vi "Measurement Done.vi"(6 "Array of Hardware":refnum<class "Hardware.lvclass">[](array[class]), 8 "error in (no error)":errorcluster, 9 "Measurement Name":string, 10 "GUID":string, 11 "Controller in":refnum<class "Controller.lvclass">) -> (0 "error out":errorcluster, 3 "Controller out":refnum<class "Controller.lvclass">)   [LabVIEW 2026, in "Controller Actor.lvlib" / "Controller.lvclass"]
uses:
  Controller.lvclass
  Hardware/Hardware.lvclass
  Hardware/Hardware.lvclass/Hardware.ctl
  <vilib>/Utility/LVClass/Get LV Class Path.vi
  <userlib>/_OpenG.lib/file/file.llb/Strip Path Extension__ogtk.vi
  <userlib>/_OpenG.lib/file/file.llb/Strip Path Extension - String__ogtk.vi
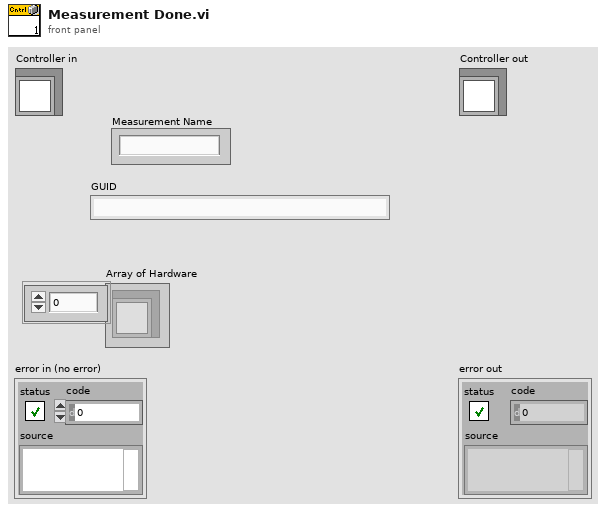
[diagram p1: front panel]
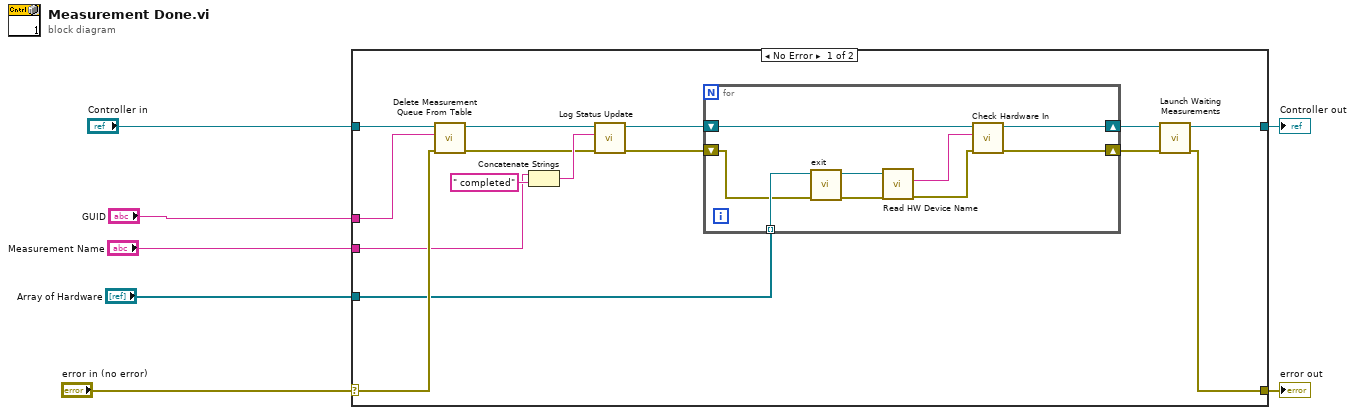
[diagram p0: block diagram]
diagram:
  n1 = case shown="No Error" "error in (no error)" {
    selector: "error in (no error)" -> [w12 w33]
    tunnel: [w11 w33] -> w6
    tunnel: [w21 w32] -> w4
    tunnel: "Controller in" -> [w15 w32]
    tunnel: "GUID" -> [w16 _]
    tunnel: "Measurement Name" -> [w10 _]
    tunnel: "Array of Hardware" -> [w9 _]
    frame No Error {
      n2 = call "Delete Measurement Queue From Table.vi"("error in (no error)"=w12, "Unique Identifier"=w16, "Controller in"=w15) -> ("error out"=w8:errorcluster, "Controller out"=w18:refnum<class "Controller.lvclass">)  [unwired: 7 in]
      n3 = Concatenate Strings(w10, " completed" ("string")) -> (w19:string)
      n4 = call-dynamic "Log Status Update.vi"("error in (no error)"=w8, "String"=w19, "Controller in"=w18) -> ("error out"=w14:errorcluster, "Controller out"=w17:refnum<class "Controller.lvclass">)  [unwired: 7 in]
      n5 = for {
        shift-right: [w30] -> w22
        shift-left: w17 -> [w31]
        shift-right: [w29] -> w13
        shift-left: w14 -> [w24]
        tunnel: w9 -> [w27] mode=indexing
        n6 = call "exit.vi"("error in (no error)"=w24, "Hardware in"=w27) -> ("error out"=w25:errorcluster, "Hardware out"=w26:refnum<class "Hardware.lvclass">)  [unwired: 8 in]
        n7 = call "Read HW Device Name.vi"("error in (no error)"=w25, "Analog in"=w26) -> ("error out"=w23:errorcluster, "Device Name"=w28:string)  [unwired: 7 in, 1 out]
        n8 = call "Check Hardware In.vi"("error in (no error)"=w23, "Hardware Name"=w28, "Controller in"=w31) -> ("error out"=w29:errorcluster, "Controller out"=w30:refnum<class "Controller.lvclass">)  [unwired: 7 in]
      }
      n9 = call "Launch Waiting Measurements.vi"("error in (no error)"=w13, "Controller in"=w22) -> ("error out"=w11:errorcluster, "Controller out"=w21:refnum<class "Controller.lvclass">)  [unwired: 8 in]
    }
    frame Error {
    }
  }
  "error out" <- w6
  "Controller out" <- w4
